vi "S2C_FORNAX_Proc_ProcessMsg.vi"(7 "Msg In":T1, 8 "Error In":errorcluster, 11 "Message":string) -> (0 "Error Out":errorcluster, 5 "Msg Out":T1)   [LabVIEW 2015]
doc: "Processes incoming Fornax messages and extracts any Viper messages."
uses:
  <vilib>/regexp/Match Regular Expression.xnode
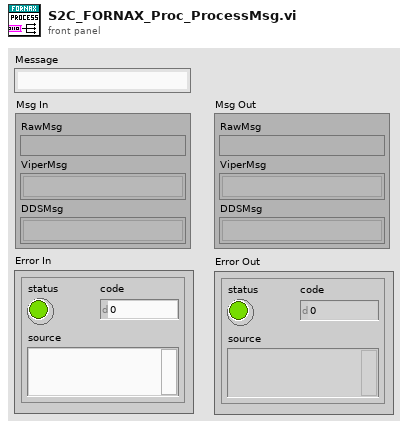
[diagram p1: front panel]
types:
  T1 = cluster{"RawMsg":string, "ViperMsg":string[], "DDSMsg":string[]}
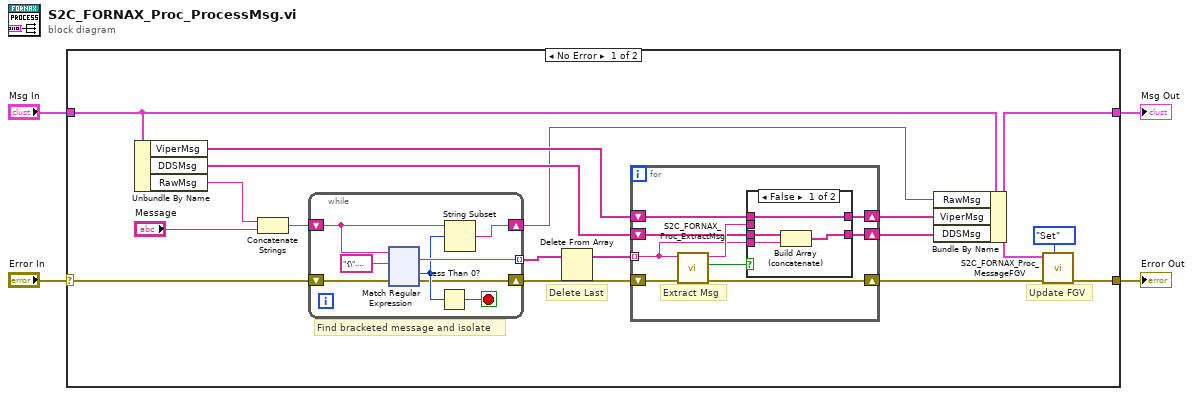
[diagram p0: block diagram]
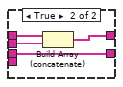
[diagram p2: hidden frame]
diagram:
  n1 = case shown="No Error" "Error In" {
    selector: "Error In" -> [w19 w159]
    tunnel: [w6 w159] -> w3
    tunnel: "Msg In" -> [w10 w158]
    tunnel: [w7 w158] -> w1
    frame No Error {
      # "Update FGV"
      # "Delete Last"
      # "Find bracketed message and isolate"
      n2 = Unbundle By Name(w10) -> ("ViperMsg"=w14:string[], "DDSMsg"=w15:string[], "RawMsg"=w20:string)
      n3 = Concatenate Strings(w20, "Message") -> (w21:string)
      n4 = while {
        shift-right: [w45] -> w11
        shift-left: w21 -> [w46]
        tunnel: [w44] -> w18 mode=indexing
        shift-right: [w40] -> w17
        shift-left: w19 -> [w41]
        stop <- w42 stop-if-true
        n5 = xnode "Match Regular Expression"("input string"=w46, "regular expression"="{\".*?}\\n|{\".*?}\\r\\n" ("format string"), "error in"=w41) -> ("whole match"=w44:string, "offset past match"=w43:i32, "error out"=w40:errorcluster)  [unwired: 3 in, 2 out]
        n6 = Less Than 0?(x=w43) -> (x < 0?=w42:bool)
        n7 = String Subset(string=w46, offset (0)=w43) -> (substring=w45:string)  [unwired: 1 in]
      }
      n8 = Delete From Array(array=w18) -> (array with subset deleted=w16:string[])  [unwired: 2 in, 1 out]
      n9 = for {
        tunnel: w16 -> [w23] mode=indexing
        shift-right: [w22] -> w8
        shift-left: w17 -> [w30]
        shift-right: [w24] -> w13
        shift-left: w14 -> [w26]
        shift-right: [w25] -> w12
        shift-left: w15 -> [w27]
        # "Extract Msg"
        n10 = call "S2C_FORNAX_Proc_ExtractMsg.vi"("Error In"=w30, "DDS Message"=w23) -> ("Error Out"=w22:errorcluster, "Found?"=w29:bool, "VIPER Message"=w28:string)  [unwired: 7 in]
        n11 = case shown="False" w29 {
          tunnel: w28 -> [_ w37]
          tunnel: w27 -> [w34 w36]
          tunnel: w26 -> [w32 w38]
          tunnel: [w33 w36] -> w25
          tunnel: [w32 w35] -> w24
          tunnel: w23 -> [w31 _]
          frame False {
            n12 = Build Array (concatenate)(w34, w31) -> (w33:string[])
          }
          frame True {
            n13 = Build Array (concatenate)(w38, w37) -> (w35:string[])
          }
        }
      }
      n14 = Bundle By Name(cluster=w10, "RawMsg"=w11, "ViperMsg"=w13, "DDSMsg"=w12) -> (w7:T1)
      n15 = call "S2C_FORNAX_Proc_MessageFGV.vi"("Action"=enum16{"Set", "Get"}."Set", "Error In"=w8, "Msg In"=w7) -> ("Error Out"=w6:errorcluster)  [unwired: 7 in, 1 out]
    }
    frame Error {
    }
  }
  "Error Out" <- w3
  "Msg Out" <- w1
